vi "Path_2_String.vi"(1 "Real Path":path) -> (0 "Path String":string)   [LabVIEW 2010]
uses:
  Globals/Constants_global.vi
  Globals/Preference_global.vi
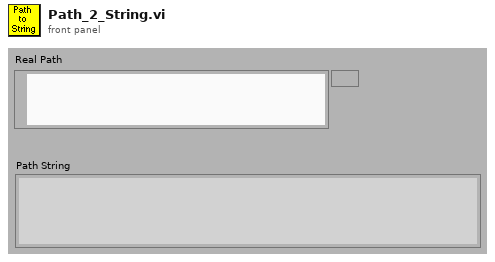
[diagram p1: front panel]
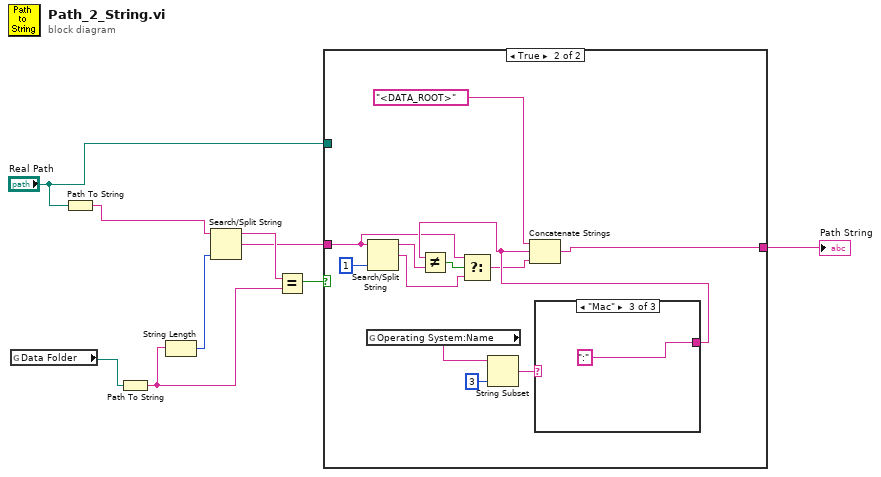
[diagram p0: block diagram]
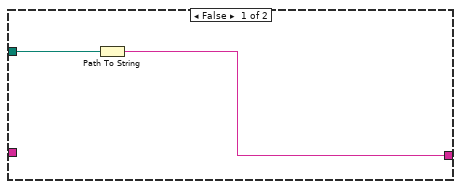
[diagram p2: hidden frame]
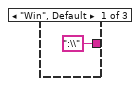
[diagram p3: hidden frame]
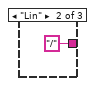
[diagram p4: hidden frame]
diagram:
  n1 = global read "Constants_global.vi" "Data Folder"() -> (w8:path)
  n2 = Path To String(path="Real Path") -> (string=w6:string)
  n3 = Path To String(path=w8) -> (string=w5:string)
  n4 = String Length(string=w5) -> (length=w7:i32)
  n5 = Search/Split String(string=w6, offset (0)=w7) -> (substring before match=w2:string, match + rest of string=w1:string)  [unwired: 1 in, 1 out]
  n6 = Equal?(x=w2, y=w5) -> (x = y?=w4:bool)
  n7 = case shown="True" w4 {
    tunnel: "Real Path" -> [w11 _]
    tunnel: [w10 w22] -> w3
    tunnel: w1 -> [_ w12]
    frame False {
      n8 = Path To String(path=w11) -> (string=w10:string)
    }
    frame True {
      n9 = global read "Preference_global.vi" "Operating System:Name"() -> (w20:string)
      n10 = Search/Split String(string=w12, offset (0)=1 ("length (rest)")) -> (substring before match=w14:string, match + rest of string=w15:string)  [unwired: 2 out]
      n11 = String Subset(string=w20, length (rest)=3 ("length (rest)")) -> (substring=w19:string)  [unwired: 1 out]
      n12 = case shown="\"Mac\"" w19 {
        tunnel: [":\\" "/" ":"] -> w17
        frame "Win", Default {
        }
        frame "Lin" {
        }
        frame "Mac" {
        }
      }
      n13 = Not Equal?(x=w17, y=w14) -> (x != y?=w16:bool)
      n14 = Select(t=w12, s=w16, f=w15) -> (s? t:f=w13:string)
      n15 = Concatenate Strings("<DATA_ROOT>", w17, w13) -> (w22:string)
    }
  }
  "Path String" <- w3
